vi "GetSTDFromLastDraw.vi"(11 "Officials Results":dbl[](array[numeric])) -> (0 "StdRes array":u64[](array[numeric]), 2 "STD":dbl, 3 "Mean":dbl format="%.2f")   [LabVIEW 2023]
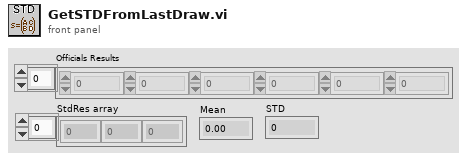
[diagram p1: front panel]
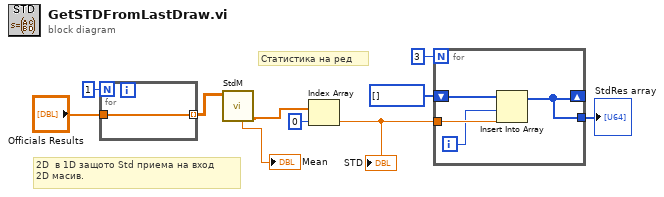
[diagram p0: block diagram]
diagram:
  # "2D  в 1D защото Std приема на вход\n2D масив."
  # "Статистика на ред"
  n1 = for {
    N: 1 -> [_]
    tunnel: "Officials Results" -> [w11]
    tunnel: [w11] -> w3 mode=indexing
  }
  n2 = call "StdM.vi"("2D in"=w3) -> ("1D Std"=w1:dbl[], "Mean from first row"=→"Mean":dbl)  [unwired: 6 in, 3 out]
  n3 = Index Array "Index Array"(array=w1, index=0) -> (element=w6:dbl)
  "STD" <- w6
  n4 = for {
    N: 3 -> [_]
    tunnel: w6 -> [w15]
    shift-right: [w12] -> _
    shift-left: u64[] [] -> [w13]
    tunnel: [w12] -> w4
    i -> [w14]
    n5 = Insert Into Array(array=w13, index=w14, new element=w15) -> (w12:u64[])
  }
  "StdRes array" <- w4
